vi "FPGAcode2.vi"() -> ()   [LabVIEW 2015]
uses:
  <vilib>/Platform/TimedLoop/XDataNode/timing_clust.ctl
  <vilib>/Platform/TimedLoop/XDataNode/nitl_modes.ctl
  <vilib>/Platform/TimedLoop/XDataNode/wakeup.ctl
  <vilib>/rvi/Emulation/niFpgaGetClockAttributes.vi
  <vilib>/rvi/Emulation/niFpgaSctlEmulationGetInTimedLoop.vi
  <vilib>/rvi/Emulation/niFpgaEmulationReportErrorSimple.vi
  <vilib>/rvi/Emulation/niFpgaProcessEmulError.vi
  <vilib>/rvi/eio/common/nirviEmuTemplateMethod_errors.vi
  <vilib>/rvi/Emulation/niFpgaCriticalErrorInLSC.vi
  <vilib>/eio/EIONode/EIONode.xnode
  <vilib>/Platform/TimedLoop/XDataNode/XDataNode.xnode
  <vilib>/Platform/TimedLoop/XDataNode/XDNodeRunTimeDep.lvlib
panel:
  out "Del Not Armed?":bool
  out "Not Armed?":bool
  in  "Reset One Shot":bool
  in  "One Shot":bool
  out "Filter 1 Detector 3 Correlation":i32
  in  "Filter 2 threshold":i32=1000
  out "Filter 2 Detector 3 Correlation":i32
  in  "Filter 1 threshold":i32=1000
  in  "Filter 3 threshold":i32=1000
  out "Filter 3 Detector 3 Correlation":i32
  in  "Filter 4 threshold":i32=1000
  out "Filter 4 Detector 3 Correlation":i32
  in  "Filter 5 threshold":i32
  out "Filter 5 Detector 3 Correlation":i32
  in  "Filter 6 threshold":i32
  out "Filter 6 Detector 3 Correlation":i32
  in  "Filter 7 threshold":i32
  out "Filter 7 Detector 3 Correlation":i32
  out "Plates":bool
  in  "High Charge Limit":i16
  in  "Low Charge Limit":i16
  in  "High Velocity Count":i32
  in  "Low Velocity Count":i32
  in  "High Mass Limit":i64
  in  "Low Mass Limit":i64
  in  "Mult1":fxp<+,16,7>
  out "Delay1":bool
  out "IO Module\\AI 0":i16
  out "IO Module\\AI 1":i16
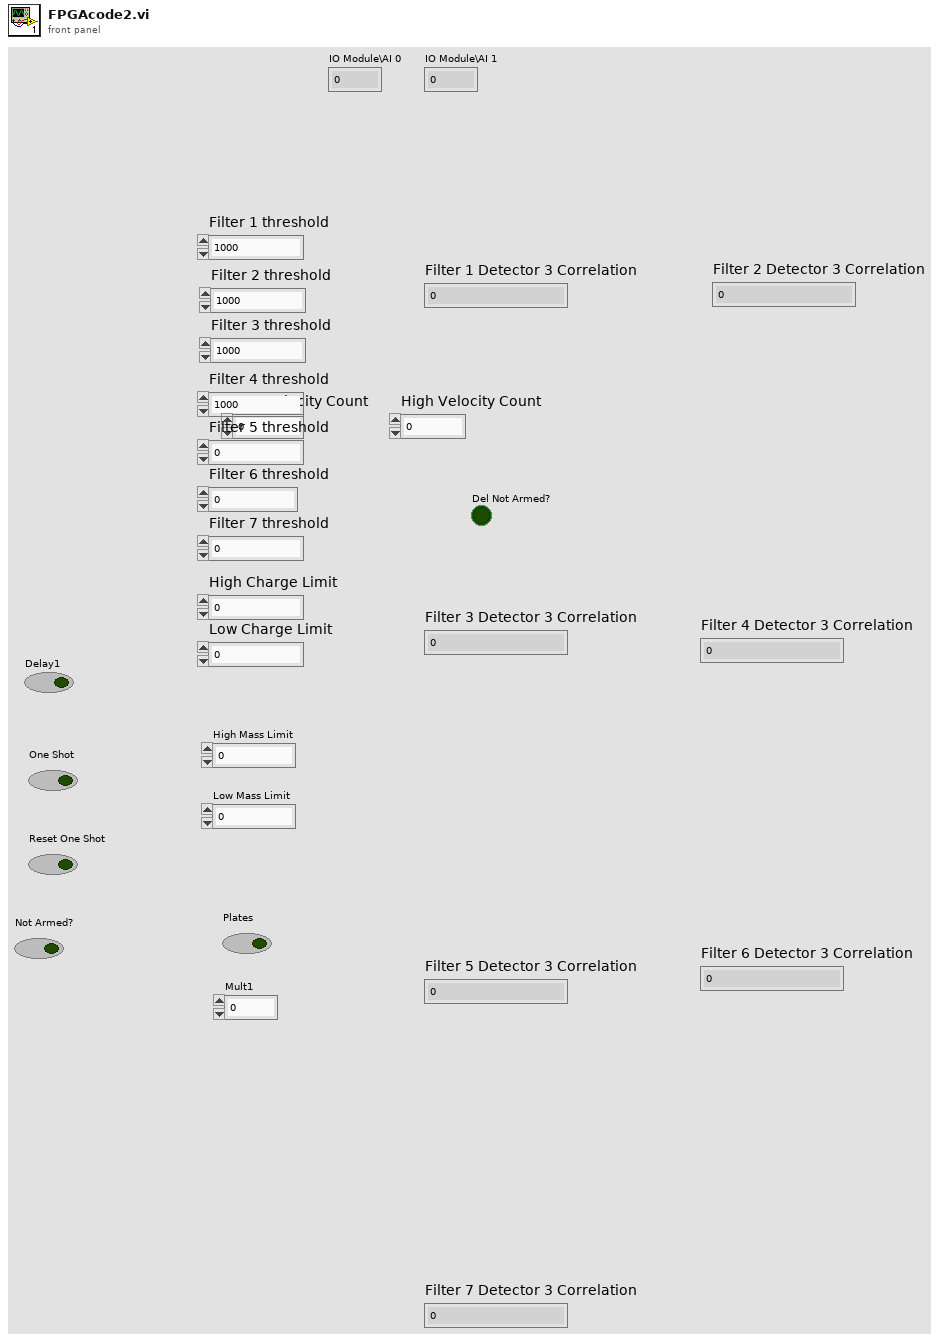
[diagram p1: front panel]
types:
  T1 = typedef "XDNodeRunTimeDep.lvlib/timing_clust.ctl" = cluster{"Expected End [f-1]":u64, "Actual End [f-1]":u64, "Finished Late? [f-1]":bool, "Expected End [i-1]":u64, "Actual End [i-1]":u64, "Finished Late? [i-1]":bool, "Expected Start [i]":u64, "Actual Start [i]":u64, "Expected Start [f]":u64, "Actual Start [f]":u64, "Source Name":string, "Structure Name":string, "Period":i64, "Deadline":i64, "Offset":i64, "Start":i64, "Priority":i32, "Timeout":i32, "Mode":T2, "Wakeup Reason":T3, "Error":errorcluster, "Source Type":string, "Secondary Source Type":string, "Global End Time":u64, "Global Start Time":u64, "Frame Duration":u64, "Iteration Duration":u64, "Assigned CPU":i32, "I/O Scan Engine Mode":u32}
  T2 = typedef "XDNodeRunTimeDep.lvlib/nitl_modes.ctl" = enum32{"No Change", "Process missed periods, maintain original phase", "Discard missed periods, maintain original phase", "Process missed periods, ignore original phase", "Discard missed periods, ignore original phase"}
  T3 = typedef "XDNodeRunTimeDep.lvlib/wakeup.ctl" = enum32{"Normal", "Aborted", "Asynchronous wakeup", "Timing source error", "Timed loop error", "Timeout"}
  T4 = cluster{"Old Average":i32, "New Average":i32, "Current State":u8, "Detector 1 Correlation":i32, "Detector 3 Correlation":i32, "Velocity Count":i32, "Detector Counter in":i32, "Timeout Count in":i32, "Measured Charge in":i32, "Filter Threshold":i32, "High Correlation in":i32, "Offset":i32, "Offset Average":i32, "Measured Velocity In":i32, "Mult Cluster":cluster{"Mult1":fxp<+,16,7>, "Mult1 Use?":bool}, "Final Delay Count In":u16, "Delay1 In":i32}
  T5 = cluster{"Separation cut off 1":i32, "Filter Number":i32, "Separation cut off 2":i32}
  T6 = cluster{"High Charge Limit":i16, "Low Charge Limit":i16, "Low Velocity Count":i32, "High Velocity Count":i32, "Low Velocity Count":i32, fxp<+,30,25>, "High Mass Limit":i64, "Low Mass Limit":i64}
  T7 = cluster{"Average Out":i32, "Next State":u8, "Velocity Count out":i32, "Detector counter out":i32, "Timeout count out":u32, "Measured Charge Out":i32, "High Correlation Out":i32, "Plates":bool, "Offset Out":i32, "Measured Velocity Out":i32, "Final Delay Count Out":u16, "Out1":bool, "Delay1":i32}
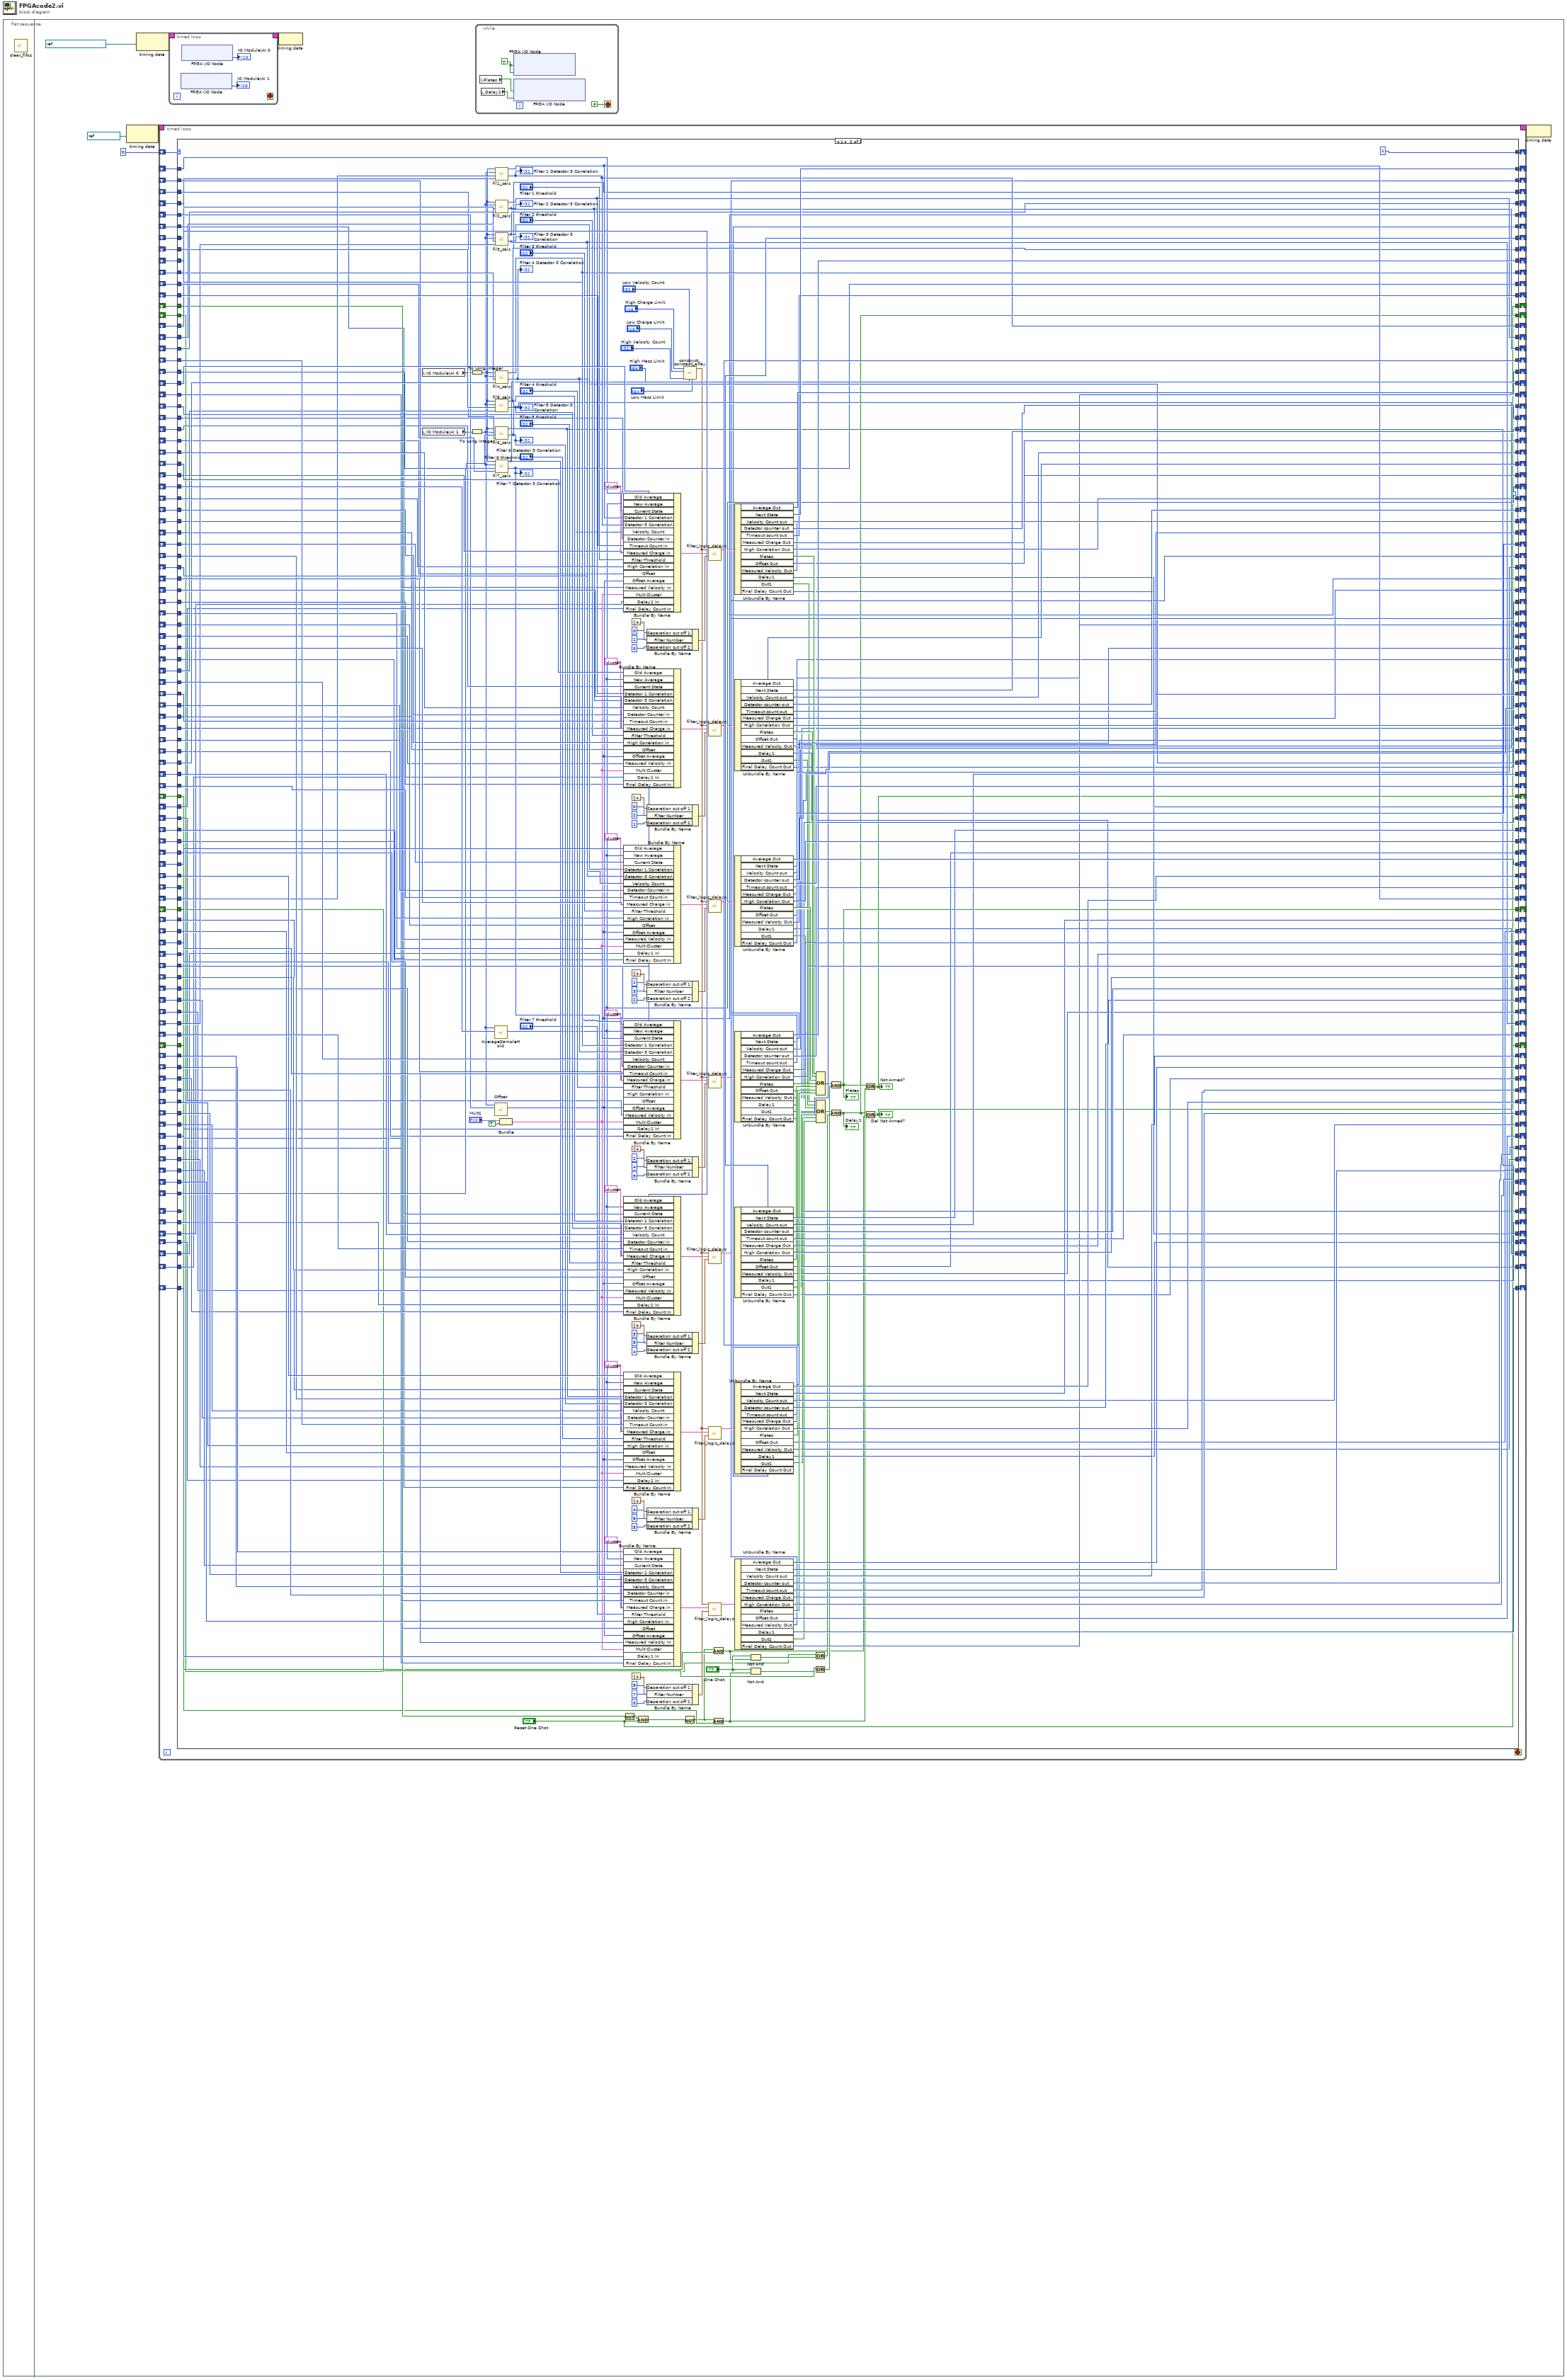
[diagram p0: block diagram]
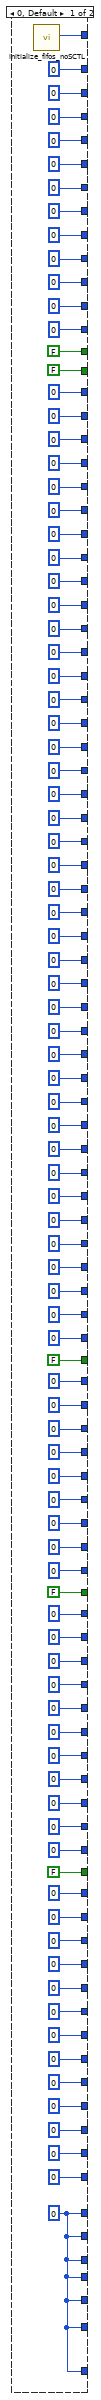
[diagram p2: hidden frame]
diagram:
  n1 = flat-sequence {
    frame #0 {
      n2 = call "clear_fifos.vi"() -> ()  [unwired: 1 in]
    }
    frame #1 {
      n3 = node-c288(refnum<k21> "26.67MHz" ("Source Name")) -> (w7:T1)
      n4 = node-c288(refnum<k21> "IO Module\\Data Clock" ("Source Name")) -> (w4:T1)
      n5 = timed-loop {
        timing: w7 -> [_]
        timing-out: [_] -> w6
        shift-right: [w211] -> _
        shift-left: _ -> [w139]
        shift-right: [w212] -> _
        shift-left: _ -> [w140]
        shift-right: [w106] -> _
        shift-left: _ -> [w141]
        shift-right: [w135] -> _
        shift-left: _ -> [w142]
        shift-right: [w105] -> _
        shift-left: _ -> [w138]
        shift-right: [w210] -> _
        shift-left: _ -> [w137]
        shift-right: [w131] -> _
        shift-left: _ -> [w134]
        shift-right: [w130] -> _
        shift-left: _ -> [w133]
        shift-right: [w104] -> _
        shift-left: _ -> [w205]
        shift-right: [w202] -> _
        shift-left: _ -> [w204]
        shift-right: [w201] -> _
        shift-left: _ -> [w203]
        shift-right: [w197] -> _
        shift-left: _ -> [w198]
        shift-right: [w126] -> _
        shift-left: _ -> [w20]
        shift-right: [w102] -> _
        shift-left: _ -> [w194]
        shift-right: [w192] -> _
        shift-left: _ -> [w193]
        shift-right: [w190] -> _
        shift-left: _ -> [w191]
        shift-right: [w101] -> _
        shift-left: _ -> [w189]
        shift-right: [w188] -> _
        shift-left: _ -> [w128]
        shift-right: [w213] -> _
        shift-left: _ -> [w215]
        shift-right: [w206] -> _
        shift-left: _ -> [w207]
        shift-right: [w127] -> _
        shift-left: _ -> [w129]
        shift-right: [w214] -> _
        shift-left: _ -> [w216]
        shift-right: [w208] -> _
        shift-left: _ -> [w209]
        shift-right: [w196] -> _
        shift-left: _ -> [w195]
        shift-right: [w92] -> _
        shift-left: _ -> [w217]
        shift-right: [w136] -> _
        shift-left: _ -> [w143]
        shift-right: [w103] -> _
        shift-left: _ -> [w199]
        shift-right: [w200] -> _
        shift-left: _ -> [w132]
        shift-right: [w187] -> _
        shift-left: _ -> [w186]
        shift-right: [w185] -> _
        shift-left: _ -> [w184]
        shift-right: [w122] -> _
        shift-left: _ -> [w124]
        shift-right: [w121] -> _
        shift-left: _ -> [w123]
        shift-right: [w100] -> _
        shift-left: _ -> [w183]
        shift-right: [w182] -> _
        shift-left: _ -> [w181]
        shift-right: [w180] -> _
        shift-left: _ -> [w179]
        shift-right: [w99] -> _
        shift-left: _ -> [w178]
        shift-right: [w177] -> _
        shift-left: _ -> [w125]
        shift-right: [w176] -> _
        shift-left: _ -> [w175]
        shift-right: [w174] -> _
        shift-left: _ -> [w173]
        shift-right: [w117] -> _
        shift-left: _ -> [w120]
        shift-right: [w116] -> _
        shift-left: _ -> [w119]
        shift-right: [w98] -> _
        shift-left: _ -> [w172]
        shift-right: [w171] -> _
        shift-left: _ -> [w170]
        shift-right: [w169] -> _
        shift-left: _ -> [w168]
        shift-right: [w97] -> _
        shift-left: _ -> [w167]
        shift-right: [w166] -> _
        shift-left: _ -> [w118]
        shift-right: [w165] -> _
        shift-left: _ -> [w163]
        shift-right: [w164] -> _
        shift-left: _ -> [w160]
        shift-right: [w113] -> _
        shift-left: _ -> [w115]
        shift-right: [w112] -> _
        shift-left: _ -> [w21]
        shift-right: [w95] -> _
        shift-left: _ -> [w162]
        shift-right: [w159] -> _
        shift-left: _ -> [w161]
        shift-right: [w158] -> _
        shift-left: _ -> [w157]
        shift-right: [w96] -> _
        shift-left: _ -> [w156]
        shift-right: [w155] -> _
        shift-left: _ -> [w114]
        shift-right: [w154] -> _
        shift-left: _ -> [w153]
        shift-right: [w152] -> _
        shift-left: _ -> [w144]
        shift-right: [w108] -> _
        shift-left: _ -> [w111]
        shift-right: [w107] -> _
        shift-left: _ -> [w110]
        shift-right: [w94] -> _
        shift-left: _ -> [w151]
        shift-right: [w150] -> _
        shift-left: _ -> [w149]
        shift-right: [w148] -> _
        shift-left: _ -> [w147]
        shift-right: [w93] -> _
        shift-left: _ -> [w146]
        shift-right: [w145] -> _
        shift-left: _ -> [w109]
        shift-right: [w90] -> _
        shift-left: i16 0 ("Output State") -> [w91]
        shift-right: [w88] -> _
        shift-left: _ -> [w89]
        shift-right: [w87] -> _
        shift-left: _ -> [w84]
        shift-right: [w85] -> _
        shift-left: _ -> [w86]
        shift-right: [w82] -> _
        shift-left: _ -> [w83]
        shift-right: [w81] -> _
        shift-left: _ -> [w80]
        shift-right: [w79] -> _
        shift-left: _ -> [w78]
        shift-right: [w77] -> _
        shift-left: _ -> [w76]
        shift-right: [w75] -> _
        shift-left: _ -> [w74]
        shift-right: [w72] -> _
        shift-left: _ -> [w73]
        shift-right: [w71] -> _
        shift-left: _ -> [w60]
        shift-right: [w70] -> _
        shift-left: _ -> [w61]
        shift-right: [w69] -> _
        shift-left: _ -> [w62]
        shift-right: [w68] -> _
        shift-left: _ -> [w63]
        shift-right: [w67] -> _
        shift-left: _ -> [w64]
        shift-right: [w66] -> _
        shift-left: _ -> [w65]
        shift-right: [w59] -> _
        shift-left: _ -> [w57]
        shift-right: [w58] -> _
        shift-left: _ -> [w56]
        shift-right: [w55] -> _
        shift-left: _ -> [w53]
        shift-right: [w54] -> _
        shift-left: _ -> [w52]
        shift-right: [w51] -> _
        shift-left: _ -> [w49]
        shift-right: [w50] -> _
        shift-left: _ -> [w48]
        shift-right: [w47] -> _
        shift-left: _ -> [w45]
        shift-right: [w46] -> _
        shift-left: _ -> [w44]
        shift-right: [w43] -> _
        shift-left: _ -> [w41]
        shift-right: [w42] -> _
        shift-left: _ -> [w40]
        shift-right: [w39] -> _
        shift-left: _ -> [w37]
        shift-right: [w38] -> _
        shift-left: _ -> [w36]
        shift-right: [w35] -> _
        shift-left: _ -> [w33]
        shift-right: [w34] -> _
        shift-left: _ -> [w32]
        shift-right: [w30] -> _
        shift-left: _ -> [w31]
        shift-right: [w29] -> _
        shift-left: _ -> [w28]
        shift-right: [w27] -> _
        shift-left: _ -> [w26]
        shift-right: [w22] -> _
        shift-left: _ -> [w25]
        shift-right: [w23] -> _
        shift-left: _ -> [w24]
        stop <- _ stop-if-true
        n6 = case shown="1" w91 {
          tunnel: w217 -> [_ w610]
          tunnel: w216 -> [_ w609]
          tunnel: w215 -> [_ w451]
          tunnel: [0 ("Average Out") w608] -> w214
          tunnel: [u16 0 ("Next State") w607] -> w213
          tunnel: [0 ("Detector counter out") w606] -> w212
          tunnel: [u32 0 ("Timeout count out") w605] -> w211
          tunnel: [0 ("High Correlation Out") w604] -> w210
          tunnel: w209 -> [_ w603]
          tunnel: [0 ("Average Out") w602] -> w208
          tunnel: w207 -> [_ w450]
          tunnel: [u16 0 ("Next State") w601] -> w206
          tunnel: w205 -> [_ w600]
          tunnel: w204 -> [_ w443]
          tunnel: w203 -> [_ w599]
          tunnel: [0 ("Detector counter out") w598] -> w202
          tunnel: [u32 0 ("Timeout count out") w597] -> w201
          tunnel: [0 ("High Correlation Out") w596] -> w200
          tunnel: w199 -> [_ w595]
          tunnel: w198 -> [_ w594]
          tunnel: [0 ("Average Out") w593] -> w197
          tunnel: [u16 0 ("Next State") w592] -> w196
          tunnel: w195 -> [_ w449]
          tunnel: w194 -> [_ w591]
          tunnel: w193 -> [_ w442]
          tunnel: [0 ("Detector counter out") w590] -> w192
          tunnel: w191 -> [_ w589]
          tunnel: [u32 0 ("Timeout count out") w588] -> w190
          tunnel: w189 -> [_ w587]
          tunnel: [0 ("High Correlation Out") w586] -> w188
          tunnel: [0 ("Average Out") w585] -> w187
          tunnel: w186 -> [_ w584]
          tunnel: [u16 0 ("Next State") w583] -> w185
          tunnel: w184 -> [_ w448]
          tunnel: w183 -> [_ w582]
          tunnel: [0 ("Detector counter out") w581] -> w182
          tunnel: w181 -> [_ w441]
          tunnel: [u32 0 ("Timeout count out") w580] -> w180
          tunnel: w179 -> [_ w579]
          tunnel: w178 -> [_ w578]
          tunnel: [0 ("High Correlation Out") w577] -> w177
          tunnel: [0 ("Average Out") w576] -> w176
          tunnel: w175 -> [_ w575]
          tunnel: [u16 0 ("Next State") w574] -> w174
          tunnel: w173 -> [_ w447]
          tunnel: w172 -> [_ w573]
          tunnel: [0 ("Detector counter out") w572] -> w171
          tunnel: w170 -> [_ w440]
          tunnel: [u32 0 ("Timeout count out") w571] -> w169
          tunnel: w168 -> [_ w570]
          tunnel: w167 -> [_ w569]
          tunnel: [0 ("High Correlation Out") w568] -> w166
          tunnel: [0 ("Average Out") w567] -> w165
          tunnel: [u16 0 ("Next State") w566] -> w164
          tunnel: w163 -> [_ w565]
          tunnel: w162 -> [_ w564]
          tunnel: w161 -> [_ w439]
          tunnel: w160 -> [_ w446]
          tunnel: [0 ("Detector counter out") w563] -> w159
          tunnel: [u32 0 ("Timeout count out") w562] -> w158
          tunnel: w157 -> [_ w561]
          tunnel: w156 -> [_ w560]
          tunnel: [0 ("High Correlation Out") w559] -> w155
          tunnel: [0 ("Average Out") w558] -> w154
          tunnel: w153 -> [_ w557]
          tunnel: [u16 0 ("Next State") w556] -> w152
          tunnel: w151 -> [_ w555]
          tunnel: [0 ("Detector counter out") w554] -> w150
          tunnel: w149 -> [_ w438]
          tunnel: [u32 0 ("Timeout count out") w553] -> w148
          tunnel: w147 -> [_ w552]
          tunnel: w146 -> [_ w551]
          tunnel: [0 ("High Correlation Out") w550] -> w145
          tunnel: w144 -> [_ w445]
          tunnel: w143 -> [_ w549]
          tunnel: w142 -> [_ w353]
          tunnel: w141 -> [_ w354]
          tunnel: w140 -> [_ w444]
          tunnel: w139 -> [_ w548]
          tunnel: w138 -> [_ w547]
          tunnel: w137 -> [_ w546]
          tunnel: [0 ("Detector 1 Correlation Out") w545] -> w136
          tunnel: [0 ("Detector 3 Correlation Out") w544] -> w135
          tunnel: w134 -> [_ w543]
          tunnel: w133 -> [_ w542]
          tunnel: w132 -> [_ w541]
          tunnel: [0 ("Detector 1 Correlation Out") w540] -> w131
          tunnel: [0 ("Detector 3 Correlation Out") w539] -> w130
          tunnel: w129 -> [_ w538]
          tunnel: w20 -> [_ w537]
          tunnel: w128 -> [_ w536]
          tunnel: [0 ("Detector 1 Correlation Out") w535] -> w127
          tunnel: [0 ("Detector 3 Correlation Out") w534] -> w126
          tunnel: w125 -> [_ w533]
          tunnel: w124 -> [_ w532]
          tunnel: w123 -> [_ w531]
          tunnel: [0 ("Detector 1 Correlation Out") w530] -> w122
          tunnel: [0 ("Detector 3 Correlation Out") w529] -> w121
          tunnel: w120 -> [_ w528]
          tunnel: w119 -> [_ w527]
          tunnel: w118 -> [_ w526]
          tunnel: [0 ("Detector 1 Correlation Out") w525] -> w117
          tunnel: [0 ("Detector 3 Correlation Out") w524] -> w116
          tunnel: w115 -> [_ w523]
          tunnel: w21 -> [_ w522]
          tunnel: w114 -> [_ w521]
          tunnel: [0 ("Detector 1 Correlation Out") w520] -> w113
          tunnel: [0 ("Detector 3 Correlation Out") w519] -> w112
          tunnel: w111 -> [_ w518]
          tunnel: w110 -> [_ w517]
          tunnel: w109 -> [_ w516]
          tunnel: [0 ("Detector 1 Correlation Out") w381] -> w108
          tunnel: [0 ("Detector 3 Correlation Out") w515] -> w107
          tunnel: [0 ("Velocity Count out") w514] -> w106
          tunnel: [0 ("Measured Charge Out") w513] -> w105
          tunnel: [0 ("Velocity Count out") w512] -> w104
          tunnel: [0 ("Measured Charge Out") w511] -> w103
          tunnel: [0 ("Velocity Count out") w510] -> w102
          tunnel: [0 ("Measured Charge Out") w509] -> w101
          tunnel: [0 ("Velocity Count out") w437] -> w100
          tunnel: [0 ("Measured Charge Out") w508] -> w99
          tunnel: [0 ("Velocity Count out") w507] -> w98
          tunnel: [0 ("Measured Charge Out") w506] -> w97
          tunnel: [0 ("Measured Charge Out") w505] -> w96
          tunnel: [0 ("Velocity Count out") w504] -> w95
          tunnel: [0 ("Velocity Count out") w503] -> w94
          tunnel: [0 ("Measured Charge Out") w502] -> w93
          tunnel: [0 ("Output New Average") w436] -> w92
          tunnel: [w310 i16 1 ("Output State")] -> w90
          tunnel: w89 -> [_ w433]
          tunnel: [0 ("Offset Out") w432] -> w88
          tunnel: [0 ("Offset Out") w431] -> w87
          tunnel: w86 -> [_ w430]
          tunnel: [0 ("Output New Average") w419] -> w85
          tunnel: w84 -> [_ w428]
          tunnel: w83 -> [_ w427]
          tunnel: [0 ("Offset Out") w426] -> w82
          tunnel: [0 ("Offset Out") w425] -> w81
          tunnel: w80 -> [_ w424]
          tunnel: [0 ("Offset Out") w423] -> w79
          tunnel: w78 -> [_ w422]
          tunnel: [0 ("Offset Out") w421] -> w77
          tunnel: w76 -> [_ w420]
          tunnel: [0 ("Offset Out") w418] -> w75
          tunnel: w74 -> [_ w417]
          tunnel: w73 -> [_ w412]
          tunnel: [0 ("Measured Velocity Out") w405] -> w72
          tunnel: [0 ("Measured Velocity Out") w404] -> w71
          tunnel: [0 ("Measured Velocity Out") w403] -> w70
          tunnel: [0 ("Measured Velocity Out") w402] -> w69
          tunnel: [0 ("Measured Velocity Out") w401] -> w68
          tunnel: [0 ("Measured Velocity Out") w400] -> w67
          tunnel: [0 ("Measured Velocity Out") w399] -> w66
          tunnel: w65 -> [_ w411]
          tunnel: w64 -> [_ w410]
          tunnel: w63 -> [_ w409]
          tunnel: w62 -> [_ w408]
          tunnel: w61 -> [_ w407]
          tunnel: w60 -> [_ w406]
          tunnel: [w223 w376] -> w59
          tunnel: [u32 0 ("Final Delay Count Out") w394] -> w58
          tunnel: w57 -> [_ w393]
          tunnel: w56 -> [_ w392]
          tunnel: [w223 w391] -> w55
          tunnel: [u32 0 ("Final Delay Count Out") w390] -> w54
          tunnel: w53 -> [_ w389]
          tunnel: w52 -> [_ w388]
          tunnel: [w223 w375] -> w51
          tunnel: [u32 0 ("Final Delay Count Out") w387] -> w50
          tunnel: w49 -> [_ w369]
          tunnel: w48 -> [_ w386]
          tunnel: [w223 w374] -> w47
          tunnel: [u32 0 ("Final Delay Count Out") w385] -> w46
          tunnel: w45 -> [_ w368]
          tunnel: w44 -> [_ w384]
          tunnel: [w223 w373] -> w43
          tunnel: [u32 0 ("Final Delay Count Out") w383] -> w42
          tunnel: w41 -> [_ w367]
          tunnel: w40 -> [_ w382]
          tunnel: [w223 w372] -> w39
          tunnel: [u32 0 ("Final Delay Count Out") w380] -> w38
          tunnel: w37 -> [_ w366]
          tunnel: w36 -> [_ w379]
          tunnel: [w223 w371] -> w35
          tunnel: [u32 0 ("Final Delay Count Out") w378] -> w34
          tunnel: w33 -> [_ w365]
          tunnel: w32 -> [_ w377]
          tunnel: w31 -> [_ w335]
          tunnel: [FALSE ("t") w348] -> w30
          tunnel: [FALSE ("f") w352] -> w29
          tunnel: w28 -> [_ w351]
          tunnel: [FALSE ("Reset One Shot") "Reset One Shot"] -> w27
          tunnel: w26 -> [_ w347]
          tunnel: w25 -> [_ w336]
          tunnel: w24 -> [_ w341]
          tunnel: [FALSE ("Delay1") w340] -> w23
          tunnel: [FALSE w338] -> w22
          frame 0, Default {
            w223 = 0
            n7 = call "initialize_fifos_noSCTL.vi"() -> ("Output State"=w310:i16)  [unwired: 11 in]
          }
          frame 1 {
            n8 = local read "IO Module\\AI 0"() -> (w435:i16)
            n9 = local read "IO Module\\AI 1"() -> (w434:i16)
            n10 = To Long Integer(number=w435) -> (32bit integer=w460:i32)
            n11 = To Long Integer(number=w434) -> (32bit integer=w429:i32)
            n12 = call "AverageSampleHold.vi"("Previous Average"=w610, "Input Value"=w429) -> ("Output New Average"=w436:i32)  [unwired: 7 in]
            n13 = call "Offset.vi"("Previous Average"=w430, "Input Value"=w429) -> ("Output New Average"=w419:i32)  [unwired: 7 in]
            n14 = call "fil1_calc.vi"("Detector 3 Correlation In"=w353, "Detector 1 Correlation In"=w549, "AI1"=w429, "AI0"=w460) -> ("Detector 3 Correlation Out"=w544:i32, "Detector 1 Correlation Out"=w545:i32)  [unwired: 4 in]
            "Filter 1 Detector 3 Correlation" <- w544
            n15 = call "fil2_calc.vi"("Detector 3 Correlation In"=w542, "Detector 1 Correlation In"=w543, "AI1"=w429, "AI0"=w460) -> ("Detector 3 Correlation Out"=w539:i32, "Detector 1 Correlation Out"=w540:i32)  [unwired: 4 in]
            "Filter 2 Detector 3 Correlation" <- w539
            n16 = call "fil3_calc.vi"("Detector 3 Correlation In"=w537, "Detector 1 Correlation In"=w538, "AI1"=w429, "AI0"=w460) -> ("Detector 3 Correlation Out"=w534:i32, "Detector 1 Correlation Out"=w535:i32)  [unwired: 4 in]
            "Filter 3 Detector 3 Correlation" <- w534
            n17 = call "fil4_calc.vi"("Detector 3 Correlation In"=w531, "Detector 1 Correlation In"=w532, "AI1"=w429, "AI0"=w460) -> ("Detector 3 Correlation Out"=w529:i32, "Detector 1 Correlation Out"=w530:i32)  [unwired: 4 in]
            "Filter 4 Detector 3 Correlation" <- w529
            n18 = call "fil5_calc.vi"("Detector 3 Correlation In"=w527, "Detector 1 Correlation In"=w528, "AI1"=w429, "AI0"=w460) -> ("Detector 3 Correlation Out"=w524:i32, "Detector 1 Correlation Out"=w525:i32)  [unwired: 4 in]
            "Filter 5 Detector 3 Correlation" <- w524
            n19 = call "fil6_calc.vi"("Detector 3 Correlation In"=w522, "Detector 1 Correlation In"=w523, "AI1"=w429, "AI0"=w460) -> ("Detector 3 Correlation Out"=w519:i32, "Detector 1 Correlation Out"=w520:i32)  [unwired: 4 in]
            "Filter 6 Detector 3 Correlation" <- w519
            n20 = call "fil7_calc.vi"("Detector 3 Correlation In"=w517, "Detector 1 Correlation In"=w518, "AI1"=w429, "AI0"=w460) -> ("Detector 3 Correlation Out"=w515:i32, "Detector 1 Correlation Out"=w381:i32)  [unwired: 4 in]
            "Filter 7 Detector 3 Correlation" <- w515
            n21 = Bundle("Mult1"="Mult1", TRUE) -> (w395:cluster{"Mult1":fxp<+,16,7>, bool})  [unwired: 1 in]
            n22 = Bundle By Name(cluster=T4 {"Old Average"=0, "New Average"=0, "Current State"=0, "Detector 1 Correlation"=0, "Detector 3 Correlation"=0, "Velocity Count"=0, "Detector Counter in"=0, "Timeout Count in"=0, "Measured Charge in"=0, "Filter Threshold"=0, "High Correlation in"=0, "Offset"=0, "Offset Average"=0, "Measured Velocity In"=0, "Mult Cluster"={"Mult1"=0.0, "Mult1 Use?"=FALSE}, "Final Delay Count In"=0, "Delay1 In"=0} ("Variables Cluster"), "Old Average"=w609, "New Average"=w436, "Current State"=w451, "Detector 1 Correlation"=w545, "Detector 3 Correlation"=w544, "Velocity Count"=w354, "Detector Counter in"=w444, "Timeout Count in"=w548, "Measured Charge in"=w547, "Filter Threshold"="Filter 1 threshold", "High Correlation in"=w546, "Offset"=w433, "Offset Average"=w419, "Measured Velocity In"=w412, "Mult Cluster"=w395, "Delay1 In"=w393, "Final Delay Count In"=w392) -> (w315:T4)
            n23 = Bundle By Name(cluster=T4 {"Old Average"=0, "New Average"=0, "Current State"=0, "Detector 1 Correlation"=0, "Detector 3 Correlation"=0, "Velocity Count"=0, "Detector Counter in"=0, "Timeout Count in"=0, "Measured Charge in"=0, "Filter Threshold"=0, "High Correlation in"=0, "Offset"=0, "Offset Average"=0, "Measured Velocity In"=0, "Mult Cluster"={"Mult1"=0.0, "Mult1 Use?"=FALSE}, "Final Delay Count In"=0, "Delay1 In"=0} ("Variables Cluster"), "Old Average"=w603, "New Average"=w436, "Current State"=w450, "Detector 1 Correlation"=w540, "Detector 3 Correlation"=w539, "Velocity Count"=w600, "Detector Counter in"=w443, "Timeout Count in"=w599, "Measured Charge in"=w595, "Filter Threshold"="Filter 2 threshold", "High Correlation in"=w541, "Offset"=w428, "Offset Average"=w419, "Measured Velocity In"=w406, "Mult Cluster"=w395, "Delay1 In"=w389, "Final Delay Count In"=w388) -> (w314:T4)
            n24 = Bundle By Name(cluster=T4 {"Old Average"=0, "New Average"=0, "Current State"=0, "Detector 1 Correlation"=0, "Detector 3 Correlation"=0, "Velocity Count"=0, "Detector Counter in"=0, "Timeout Count in"=0, "Measured Charge in"=0, "Filter Threshold"=0, "High Correlation in"=0, "Offset"=0, "Offset Average"=0, "Measured Velocity In"=0, "Mult Cluster"={"Mult1"=0.0, "Mult1 Use?"=FALSE}, "Final Delay Count In"=0, "Delay1 In"=0} ("Variables Cluster"), "Old Average"=w594, "New Average"=w436, "Current State"=w449, "Detector 1 Correlation"=w535, "Detector 3 Correlation"=w534, "Velocity Count"=w591, "Detector Counter in"=w442, "Timeout Count in"=w589, "Measured Charge in"=w587, "Filter Threshold"="Filter 3 threshold", "High Correlation in"=w536, "Offset"=w427, "Offset Average"=w419, "Measured Velocity In"=w407, "Mult Cluster"=w395, "Delay1 In"=w369, "Final Delay Count In"=w386) -> (w313:T4)
            n25 = Bundle By Name(cluster=T4 {"Old Average"=0, "New Average"=0, "Current State"=0, "Detector 1 Correlation"=0, "Detector 3 Correlation"=0, "Velocity Count"=0, "Detector Counter in"=0, "Timeout Count in"=0, "Measured Charge in"=0, "Filter Threshold"=0, "High Correlation in"=0, "Offset"=0, "Offset Average"=0, "Measured Velocity In"=0, "Mult Cluster"={"Mult1"=0.0, "Mult1 Use?"=FALSE}, "Final Delay Count In"=0, "Delay1 In"=0} ("Variables Cluster"), "Old Average"=w584, "New Average"=w436, "Current State"=w448, "Detector 1 Correlation"=w530, "Detector 3 Correlation"=w529, "Velocity Count"=w582, "Detector Counter in"=w441, "Timeout Count in"=w579, "Measured Charge in"=w578, "Filter Threshold"="Filter 4 threshold", "High Correlation in"=w533, "Offset"=w424, "Offset Average"=w419, "Measured Velocity In"=w408, "Mult Cluster"=w395, "Delay1 In"=w368, "Final Delay Count In"=w384) -> (w312:T4)
            n26 = Bundle By Name(cluster=T4 {"Old Average"=0, "New Average"=0, "Current State"=0, "Detector 1 Correlation"=0, "Detector 3 Correlation"=0, "Velocity Count"=0, "Detector Counter in"=0, "Timeout Count in"=0, "Measured Charge in"=0, "Filter Threshold"=0, "High Correlation in"=0, "Offset"=0, "Offset Average"=0, "Measured Velocity In"=0, "Mult Cluster"={"Mult1"=0.0, "Mult1 Use?"=FALSE}, "Final Delay Count In"=0, "Delay1 In"=0} ("Variables Cluster"), "Old Average"=w575, "New Average"=w436, "Current State"=w447, "Detector 1 Correlation"=w525, "Detector 3 Correlation"=w524, "Velocity Count"=w573, "Detector Counter in"=w440, "Timeout Count in"=w570, "Measured Charge in"=w569, "Filter Threshold"="Filter 5 threshold", "High Correlation in"=w526, "Offset"=w422, "Offset Average"=w419, "Measured Velocity In"=w409, "Mult Cluster"=w395, "Delay1 In"=w367, "Final Delay Count In"=w382) -> (w317:T4)
            n27 = Bundle By Name(cluster=T4 {"Old Average"=0, "New Average"=0, "Current State"=0, "Detector 1 Correlation"=0, "Detector 3 Correlation"=0, "Velocity Count"=0, "Detector Counter in"=0, "Timeout Count in"=0, "Measured Charge in"=0, "Filter Threshold"=0, "High Correlation in"=0, "Offset"=0, "Offset Average"=0, "Measured Velocity In"=0, "Mult Cluster"={"Mult1"=0.0, "Mult1 Use?"=FALSE}, "Final Delay Count In"=0, "Delay1 In"=0} ("Variables Cluster"), "Old Average"=w565, "New Average"=w436, "Current State"=w446, "Detector 1 Correlation"=w520, "Detector 3 Correlation"=w519, "Velocity Count"=w564, "Detector Counter in"=w439, "Timeout Count in"=w561, "Measured Charge in"=w560, "Filter Threshold"="Filter 6 threshold", "High Correlation in"=w521, "Offset"=w420, "Offset Average"=w419, "Measured Velocity In"=w410, "Mult Cluster"=w395, "Delay1 In"=w366, "Final Delay Count In"=w379) -> (w316:T4)
            n28 = Bundle By Name(cluster=T4 {"Old Average"=0, "New Average"=0, "Current State"=0, "Detector 1 Correlation"=0, "Detector 3 Correlation"=0, "Velocity Count"=0, "Detector Counter in"=0, "Timeout Count in"=0, "Measured Charge in"=0, "Filter Threshold"=0, "High Correlation in"=0, "Offset"=0, "Offset Average"=0, "Measured Velocity In"=0, "Mult Cluster"={"Mult1"=0.0, "Mult1 Use?"=FALSE}, "Final Delay Count In"=0, "Delay1 In"=0} ("Variables Cluster"), "Old Average"=w557, "New Average"=w436, "Current State"=w445, "Detector 1 Correlation"=w381, "Detector 3 Correlation"=w515, "Velocity Count"=w555, "Detector Counter in"=w438, "Timeout Count in"=w552, "Measured Charge in"=w551, "Filter Threshold"="Filter 7 threshold", "High Correlation in"=w516, "Offset"=w417, "Offset Average"=w419, "Measured Velocity In"=w411, "Mult Cluster"=w395, "Delay1 In"=w365, "Final Delay Count In"=w377) -> (w311:T4)
            n29 = Not(x=w347) -> (.not. x?=w333:bool)
            n30 = And(x=w333, y="Reset One Shot") -> (x .and. y?=w332:bool)
            n31 = Bundle By Name(cluster=T5 {"Separation cut off 1"=4, "Filter Number"=5, "Separation cut off 2"=6} ("Filter Specific Constants"), "Separation cut off 1"=0, "Filter Number"=1, "Separation cut off 2"=0) -> (w491:T5)
            n32 = Bundle By Name(cluster=T5 {"Separation cut off 1"=4, "Filter Number"=5, "Separation cut off 2"=6} ("Filter Specific Constants"), "Separation cut off 1"=0, "Filter Number"=2, "Separation cut off 2"=1) -> (w493:T5)
            n33 = Bundle By Name(cluster=T5 {"Separation cut off 1"=4, "Filter Number"=5, "Separation cut off 2"=6} ("Filter Specific Constants"), "Separation cut off 1"=1, "Filter Number"=3, "Separation cut off 2"=2) -> (w489:T5)
            n34 = Bundle By Name(cluster=T5 {"Separation cut off 1"=4, "Filter Number"=5, "Separation cut off 2"=6} ("Filter Specific Constants"), "Separation cut off 1"=2, "Filter Number"=4, "Separation cut off 2"=3) -> (w487:T5)
            n35 = Bundle By Name(cluster=T5 {"Separation cut off 1"=4, "Filter Number"=5, "Separation cut off 2"=6} ("Filter Specific Constants"), "Separation cut off 1"=3, "Filter Number"=5, "Separation cut off 2"=4) -> (w485:T5)
            n36 = Bundle By Name(cluster=T5 {"Separation cut off 1"=4, "Filter Number"=5, "Separation cut off 2"=6} ("Filter Specific Constants"), "Separation cut off 1"=4, "Filter Number"=6, "Separation cut off 2"=5) -> (w483:T5)
            n37 = Bundle By Name(cluster=T5 {"Separation cut off 1"=4, "Filter Number"=5, "Separation cut off 2"=6} ("Filter Specific Constants"), "Separation cut off 1"=5, "Filter Number"=7, "Separation cut off 2"=0) -> (w356:T5)
            n38 = Not(x=w332) -> (.not. x?=w331:bool)
            n39 = call "construct_constant_array.vi"("Low Mass Limit"="Low Mass Limit", "High Mass Limit"="High Mass Limit", "Low Velocity Count"="Low Velocity Count", "High Velocity Count"="High Velocity Count", "Low Charge Limit"="Low Charge Limit", "High Charge Limit"="High Charge Limit") -> ("constants cluster"=w396:T6)  [unwired: 5 in]
            n40 = call "filter_logic_delays.vi"("Filter Specific Constants"=w491, "Variables Cluster"=w315, "controls cluster"=w396) -> ("Output Cluster"=w490:T7)  [unwired: 8 in]
            n41 = call "filter_logic_delays.vi"("Filter Specific Constants"=w493, "Variables Cluster"=w314, "controls cluster"=w396) -> ("Output Cluster"=w500:T7)  [unwired: 8 in]
            n42 = call "filter_logic_delays.vi"("Filter Specific Constants"=w489, "Variables Cluster"=w313, "controls cluster"=w396) -> ("Output Cluster"=w488:T7)  [unwired: 8 in]
            n43 = call "filter_logic_delays.vi"("Filter Specific Constants"=w487, "Variables Cluster"=w312, "controls cluster"=w396) -> ("Output Cluster"=w486:T7)  [unwired: 8 in]
            n44 = call "filter_logic_delays.vi"("Filter Specific Constants"=w485, "Variables Cluster"=w317, "controls cluster"=w396) -> ("Output Cluster"=w484:T7)  [unwired: 8 in]
            n45 = call "filter_logic_delays.vi"("Filter Specific Constants"=w483, "Variables Cluster"=w316, "controls cluster"=w396) -> ("Output Cluster"=w482:T7)  [unwired: 8 in]
            n46 = call "filter_logic_delays.vi"("Filter Specific Constants"=w356, "Variables Cluster"=w311, "controls cluster"=w396) -> ("Output Cluster"=w492:T7)  [unwired: 8 in]
            n47 = And(x=w331, y=w336) -> (x .and. y?=w339:bool)
            n48 = And(x=w331, y=w335) -> (x .and. y?=w349:bool)
            n49 = Unbundle By Name(w490) -> ("Average Out"=w608:i32, "Next State"=w607:u8, "Velocity Count out"=w514:i32, "Detector counter out"=w606:i32, "Timeout count out"=w605:u32, "Measured Charge Out"=w513:i32, "High Correlation Out"=w604:i32, "Plates"=w458:bool, "Offset Out"=w432:i32, "Measured Velocity Out"=w405:i32, "Delay1"=w376:i32, "Out1"=w370:bool, "Final Delay Count Out"=w394:u16)
            n50 = Unbundle By Name(w500) -> ("Average Out"=w602:i32, "Next State"=w601:u8, "Velocity Count out"=w512:i32, "Detector counter out"=w598:i32, "Timeout count out"=w597:u32, "Measured Charge Out"=w511:i32, "High Correlation Out"=w596:i32, "Plates"=w457:bool, "Offset Out"=w431:i32, "Measured Velocity Out"=w404:i32, "Delay1"=w391:i32, "Out1"=w327:bool, "Final Delay Count Out"=w390:u16)
            n51 = Unbundle By Name(w488) -> ("Average Out"=w593:i32, "Next State"=w592:u8, "Velocity Count out"=w510:i32, "Detector counter out"=w590:i32, "Timeout count out"=w588:u32, "Measured Charge Out"=w509:i32, "High Correlation Out"=w586:i32, "Plates"=w456:bool, "Offset Out"=w426:i32, "Measured Velocity Out"=w403:i32, "Delay1"=w375:i32, "Out1"=w330:bool, "Final Delay Count Out"=w387:u16)
            n52 = Unbundle By Name(w486) -> ("Average Out"=w585:i32, "Next State"=w583:u8, "Velocity Count out"=w437:i32, "Detector counter out"=w581:i32, "Timeout count out"=w580:u32, "Measured Charge Out"=w508:i32, "High Correlation Out"=w577:i32, "Plates"=w455:bool, "Offset Out"=w425:i32, "Measured Velocity Out"=w402:i32, "Delay1"=w374:i32, "Out1"=w329:bool, "Final Delay Count Out"=w385:u16)
            n53 = Unbundle By Name(w484) -> ("Average Out"=w576:i32, "Next State"=w574:u8, "Velocity Count out"=w507:i32, "Detector counter out"=w572:i32, "Timeout count out"=w571:u32, "Measured Charge Out"=w506:i32, "High Correlation Out"=w568:i32, "Plates"=w454:bool, "Offset Out"=w423:i32, "Measured Velocity Out"=w401:i32, "Delay1"=w373:i32, "Out1"=w328:bool, "Final Delay Count Out"=w383:u16)
            n54 = Unbundle By Name(w482) -> ("Average Out"=w567:i32, "Next State"=w566:u8, "Velocity Count out"=w504:i32, "Detector counter out"=w563:i32, "Timeout count out"=w562:u32, "Measured Charge Out"=w505:i32, "High Correlation Out"=w559:i32, "Plates"=w453:bool, "Offset Out"=w421:i32, "Measured Velocity Out"=w400:i32, "Delay1"=w372:i32, "Out1"=w325:bool, "Final Delay Count Out"=w380:u16)
            n55 = Unbundle By Name(w492) -> ("Average Out"=w558:i32, "Next State"=w556:u8, "Velocity Count out"=w503:i32, "Detector counter out"=w554:i32, "Timeout count out"=w553:u32, "Measured Charge Out"=w502:i32, "High Correlation Out"=w550:i32, "Plates"=w452:bool, "Offset Out"=w418:i32, "Measured Velocity Out"=w399:i32, "Delay1"=w371:i32, "Out1"=w326:bool, "Final Delay Count Out"=w378:u16)
            n56 = Not And(1:w339, 2:"One Shot") -> (0:w342:bool)
            n57 = Not And(1:w349, 2:"One Shot") -> (0:w344:bool)
            n58 = Or(x=w341, y=w342) -> (x .or. y?=w346:bool)
            n59 = Or(x=w351, y=w344) -> (x .or. y?=w350:bool)
            n60 = Compound Arithmetic op=OR(w458, w457, w456, w455, w454, w453, w452) -> (w355:bool)
            n61 = Compound Arithmetic op=OR(w370, w327, w330, w329, w328, w325, w326) -> (w345:bool)
            n62 = And(x=w355, y=w350) -> (x .and. y?=w352:bool)
            "Plates" <- w352
            n63 = And(x=w345, y=w346) -> (x .and. y?=w340:bool)
            "Delay1" <- w340
            n64 = Or(x=w352, y=w349) -> (x .or. y?=w348:bool)
            "Not Armed?" <- w348
            n65 = Or(x=w340, y=w339) -> (x .or. y?=w338:bool)
            "Del Not Armed?" <- w338
          }
        }
      }
      n66 = timed-loop {
        timing: w4 -> [_]
        timing-out: [_] -> w3
        stop <- _ stop-if-true
        n67 = xnode "FPGA I/O Node"() -> ("IO Module\\AI 1"=→"IO Module\\AI 1":i16)  [unwired: 1 in, 1 out]
        n68 = xnode "FPGA I/O Node"() -> ("IO Module\\AI 0"=→"IO Module\\AI 0":i16)  [unwired: 1 in, 1 out]
      }
      n69 = node-c288(w3) -> ()
      n70 = while {
        stop <- FALSE stop-if-true
        w19 = TRUE ("IO Module\\PFI Enable")
        n71 = local read "Plates"() -> (w16:bool)
        n72 = local read "Delay1"() -> (w17:bool)
        n73 = xnode "FPGA I/O Node"("IO Module\\PFI 0 WE"=w19, "IO Module\\PFI 1 WE"=w19) -> ()  [unwired: 2 in, 2 out]
        n74 = xnode "FPGA I/O Node"("IO Module\\PFI 0 Wr Data"=w16, "IO Module\\PFI 1 Wr Data"=w17) -> ()  [unwired: 2 in, 2 out]
      }
      n75 = node-c288(w6) -> ()
    }
  }
